vi "PSD2.vi"(8 "error in (no error)":errorcluster, 9 "axis":string, 10 "data":dbl[](array[numeric]), 11 "Refnum in":refnum<k35>) -> (0 "error out":errorcluster, 2 "Array":cluster{dbl, dbl, dbl[]}[](array[cluster]), 3 "Refnum out":refnum<k35>)   [LabVIEW 2019]
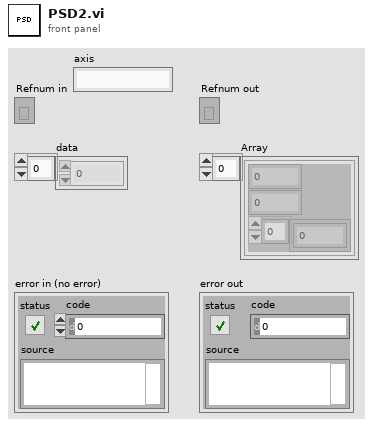
[diagram p1: front panel]
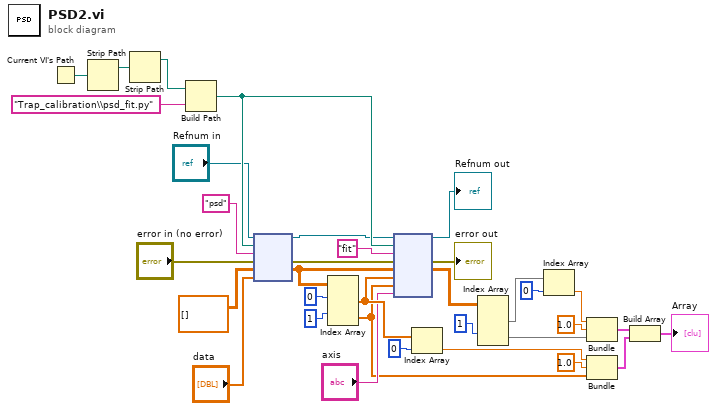
[diagram p0: block diagram]
diagram:
  n1 = Current VI's Path() -> (path=w8:path)
  n2 = Strip Path(path=w8) -> (stripped path=w2:path)  [unwired: 1 out]
  n3 = Strip Path(path=w2) -> (stripped path=w1:path)  [unwired: 1 out]
  n4 = Build Path(base path=w1, name or relative path="Trap_calibration\\psd_fit.py") -> (appended path=w15:path)
  n5 = node("Refnum in", w15, "psd" ("function name"), "error in (no error)", dbl[][] [], "data") -> (w11:refnum<k35>, w13:errorcluster, w16:dbl[][])  [unwired: 1 in, 2 out]
  n6 = Index Array(array=w16, index (row) #1=0 ("index (row)"), index (row) #2=1 ("index (row)")) -> (element #1=w23:dbl[], element #2=w17:dbl[])  [unwired: 2 in]
  n7 = node(w11, w15, "fit" ("function name"), w13, w16, w23, w17, "axis") -> (→"Refnum out":refnum<k35>, →"error out":errorcluster, w20:dbl[][])  [unwired: 3 in, 2 out]
  n8 = Index Array(array=w23, index=0) -> (element=w25:dbl)
  n9 = Index Array(array=w20, index (row) #2=1 ("index (row)")) -> (element #1=w26:dbl[], element #2=w21:dbl[])  [unwired: 3 in]
  n10 = Index Array(array=w26, index=0) -> (element=w29:dbl)
  n11 = Bundle(w29, 1.0, w21) -> (w32:cluster{dbl, dbl, dbl[]})  [unwired: 1 in]
  n12 = Bundle(w25, 1.0, w17) -> (w33:cluster{dbl, dbl, dbl[]})  [unwired: 1 in]
  n13 = Build Array(w32, w33) -> (→"Array":cluster{dbl, dbl, dbl[]}[])
